vi "Custom Probes.vi"() -> ()   [LabVIEW 2023]
doc: "This example demonstrates custom probes with LabVIEW classes.\n\nRefer to the LabVIEW Help for more information about LabVIEW object-oriented programming."
uses:
  Vehicle/Vehicle.lvclass
  Truck/Truck.lvclass
panel:
  out "truck":refnum<class "Truck.lvclass">
  out "vehicle":refnum<class "Vehicle.lvclass">
  # "Overview: Demonstrates the use of generic and custom probes with LabVIEW classes.\nInstructions:\nOpen the block diagram and follow the instructions there."
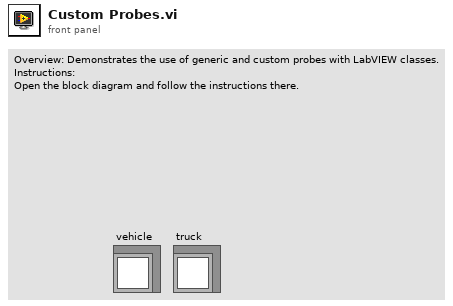
[diagram p1: front panel]
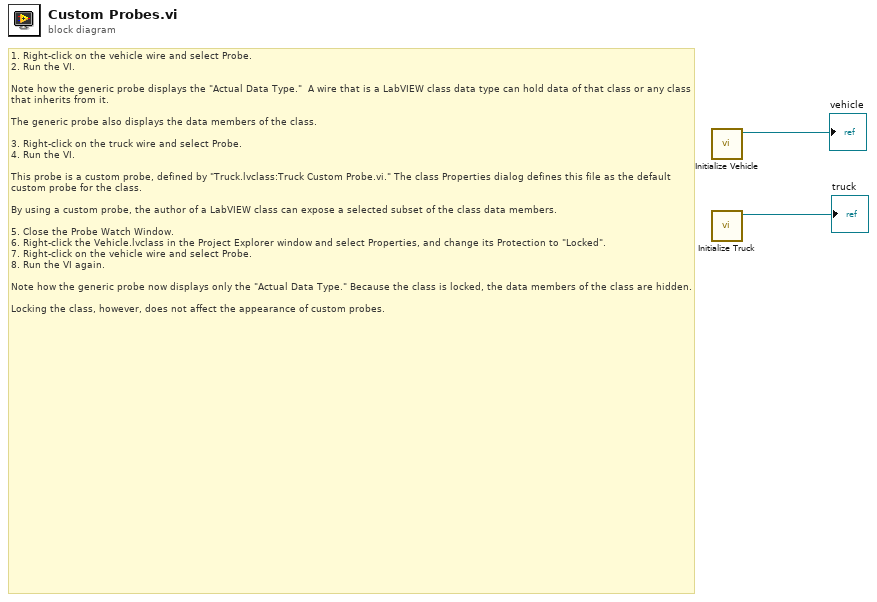
[diagram p0: block diagram]
diagram:
  # "1. Right-click on the vehicle wire and select Probe.\n2. Run the VI.\n\nNote how the generic probe displays the \"Actual Data Type.\"  A wire that is a LabVIEW class data type can hold data of that class or any class that inherits from it.\n\nThe generic probe also displays the data members of the class.\n\n3. Right-click on the truck wire and select Probe.\n4. Run the VI.\n\nThis probe is a custom probe, defined by \"Truck.lvclass:Truck Custom Probe.vi.\" The class Properties dialog defines this file as the default custom probe for the class.\n\nBy using a custom probe, the author of a LabVIEW class can expose a selected subset of the class data members.\n\n5. Close the Probe Watch Window.\n6. Right-click the Vehicle.lvclass in the Project Explorer window and select Properties, and change its Protection to \"Locked\".\n7. Right-click on the vehicle wire and select Probe.\n8. Run the VI again.\n\nNote how the generic probe now displays only the \"Actual Data Type.\" Because the class is locked, the data members of the class are hidden.\n\nLocking the class, however, does not affect the appearance of custom probes."
  n1 = call "Initialize Vehicle.vi"() -> ("vehicle out"=→"vehicle":refnum<class "Vehicle.lvclass">)  [unwired: 11 in]
  n2 = call "Initialize Truck.vi"() -> ("truck out"=→"truck":refnum<class "Truck.lvclass">)  [unwired: 11 in]
